vi "AutoMacroEngineALB.vi"(11 "Macro":T1 {"Sequence"."Axes 2"."Switch" format="%#_4g"; "Sequence"."Axes 2"."Axis 2" format="%#_4g"; "Sequence"."Axes 2"."Axis 1" format="%#_4g"; "Sequence"."Axes 2"."Axis 0" format="%#_4g"; "Sequence"."Axes 1"."Slider" format="%#_4g"; "Sequence"."Axes 1"."Axis 2" format="%#_4g"; "Sequence"."Axes 1"."Axis 1" format="%#_4g"; "Sequence"."Axes 1"."Axis 0" format="%#_4g"}) -> ()   [LabVIEW 2017]
uses:
  CtrlRefs/MacrosALB.ctl
  CtrlRefs/JoyStick1ALB.ctl
  CtrlRefs/JoyStick1ALV(Analog).ctl
  CtrlRefs/JoyStick2ALB.ctl
  CtrlRefs/JoyStick2ALB(Analog).ctl
  <vilib>/Rock Robotics/Network Tables/NT Write Number.vi
  <vilib>/Rock Robotics/Network Tables/NT Write Numeric Array.vi
  Support Code/Gyro/Gyro_TypeDef.ctl
panel:
  out "error out":errorcluster
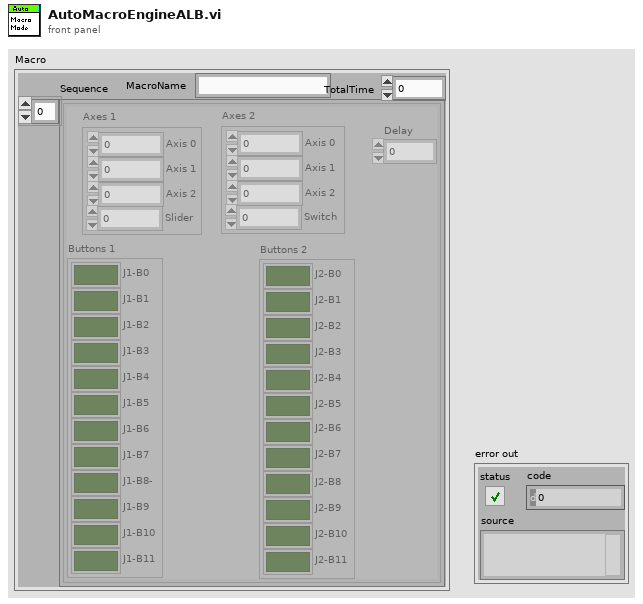
[diagram p1: front panel]
types:
  T1 = typedef "MacrosALB.ctl" = cluster{"MacroName":string, "Sequence":cluster{"Buttons 1":T2, "Axes 1":T3, "Buttons 2":T4, "Axes 2":T5, "Delay":u32}[], "TotalTime":u32}
  T2 = typedef "JoyStick1ALB.ctl" = cluster{"J1-B0":bool, "J1-B1":bool, "J1-B2":bool, "J1-B3":bool, "J1-B4":bool, "J1-B5":bool, "J1-B6":bool, "J1-B7":bool, "J1-B8-":bool, "J1-B9":bool, "J1-B10":bool, "J1-B11":bool}
  T3 = typedef "JoyStick1ALV(Analog).ctl" = cluster{"Axis 0":dbl, "Axis 1":dbl, "Axis 2":dbl, "Slider":dbl}
  T4 = typedef "JoyStick2ALB.ctl" = cluster{"J2-B0":bool, "J2-B1":bool, "J2-B2":bool, "J2-B3":bool, "J2-B4":bool, "J2-B5":bool, "J2-B6":bool, "J2-B7":bool, "J2-B8":bool, "J2-B9":bool, "J2-B10":bool, "J2-B11":bool}
  T5 = typedef "JoyStick2ALB(Analog).ctl" = cluster{"Axis 0":dbl, "Axis 1":dbl, "Axis 2":dbl, "Switch":dbl}
  T6 = cluster{"Buttons 1":T2, "Axes 1":T3, "Buttons 2":T4, "Axes 2":T5, "Delay":u32}[]
  T7 = cluster{"Output":dbl, "Output":dbl, "Output":dbl, "Output":dbl}
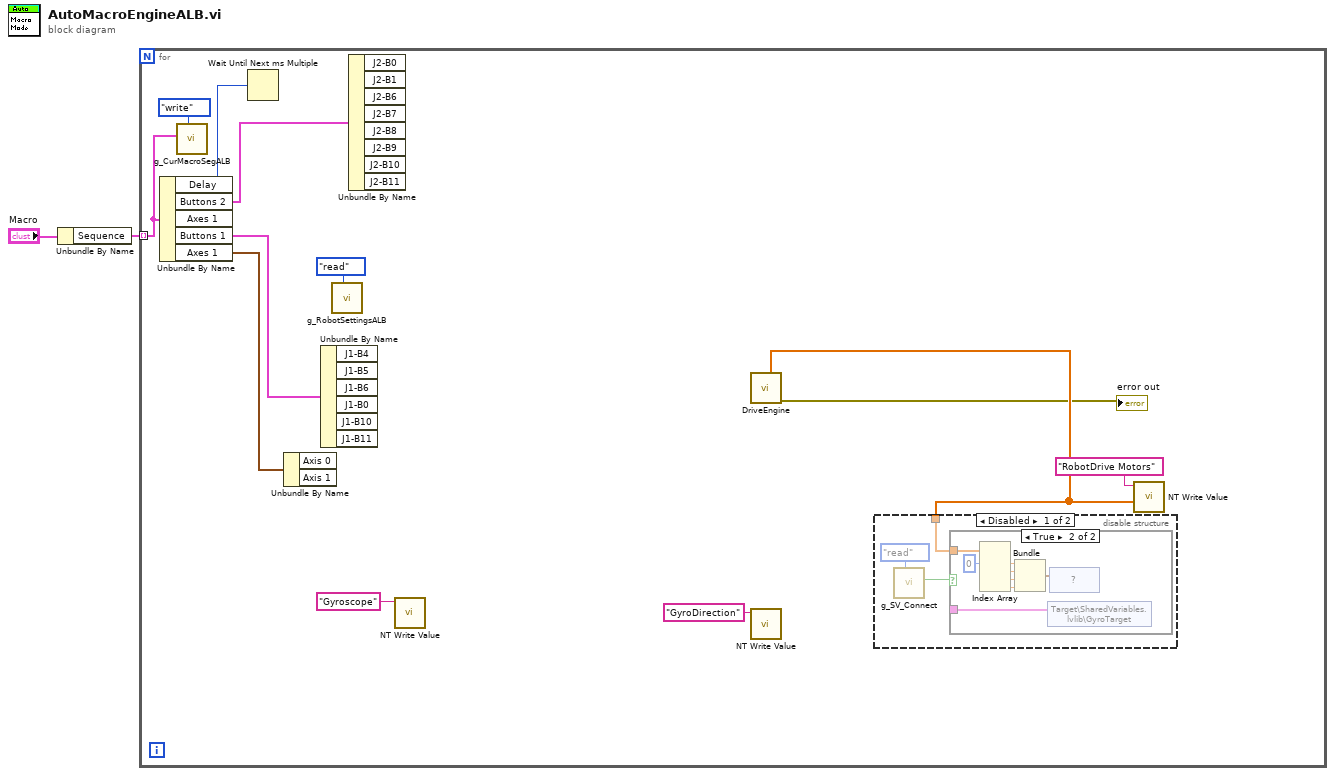
[diagram p0: block diagram]
diagram:
  n1 = Unbundle By Name("Macro") -> ("Sequence"=w1:T6)
  n2 = for {
    tunnel: w1 -> [w5] mode=indexing
    n3 = Unbundle By Name(w5) -> ("Delay"=w14:u32, "Buttons 2"=w11:T4, "Buttons 1"=w12:T2, "Axes 1"=w10:T3)  [unwired: 1 out]
    n4 = call "g_CurMacroSegALB.vi"("Action"=enum16{"read", "write"}."write", "Seg in"=w5) -> ()  [unwired: 9 in, 1 out]
    n5 = Wait Until Next ms Multiple(millisecond multiple=w14) -> ()  [unwired: 1 out]
    n6 = Unbundle By Name(w10) -> ()  [unwired: 2 out]
    n7 = Unbundle By Name(w12) -> ()  [unwired: 6 out]
    n8 = call "g_RobotSettingsALB.vi"("Action"=enum16{"read", "write"}."read") -> ()  [unwired: 10 in, 1 out]
    n9 = Unbundle By Name(w11) -> ()  [unwired: 8 out]
    n10 = call-poly <vilib>:"NT Write Value.vi"("Name"="Gyroscope") -> ()  [unwired: 10 in, 1 out]
    n11 = call "DriveEngine.vi"() -> ("error out"=→"error out":errorcluster, "Motor Values"=w4:dbl[])  [unwired: 7 in, 3 out]
    n12 = call-poly <vilib>:"NT Write Value.vi"("Name"="GyroDirection") -> ()  [unwired: 10 in, 1 out]
    n13 = disable-structure shown="Disabled" {
      disable-tunnel: w4 -> [w15 _]
      frame Disabled {
        n14 = call "g_SV_Connect.vi"("Action"=enum16{"read", "write"}."read") -> ("Connected"=w16:bool)  [unwired: 10 in]
        n15 = case shown="True" w16 {
          tunnel: w15 -> [_ w19]
          tunnel: _ -> [_ w18]
          frame False {
          }
          frame True {
            n16 = Index Array(array=w19, index #1=0 ("index")) -> (element #1=w21:dbl, element #2=w22:dbl, element #3=w23:dbl, element #4=w24:dbl)  [unwired: 3 in]
            n17 = Bundle("Output"=w21, "Output"=w22, "Output"=w23, "Output"=w24) -> (w25:T7)  [unwired: 1 in]
            n18 = shared-variable "Target\\SharedVariables.lvlib\\GyroTarget"(w18) -> ()  [unwired: 1 in, 1 out]
            n19 = shared-variable "?"(w25) -> ()  [unwired: 1 in, 1 out]
          }
        }
      }
      frame Enabled {
      }
    }
    n20 = call-poly <vilib>:"NT Write Value.vi"("Numeric Array"=w4, "Name"="RobotDrive Motors") -> ()  [unwired: 9 in, 1 out]
  }
